vi "1022test.vi"() -> ()   [LabVIEW 2019]
panel:
  out "Read Buffer":string
  in  "Timeout":u32=1000
  in  "Remote Mode":u16(ring) items=["USB", "RS232", "GPIB"]
  out "Serial Versions":string
  in  "Baud rate (921600)":u32=921600
  in  "VISA resource name":refnum<visa-resource-name>
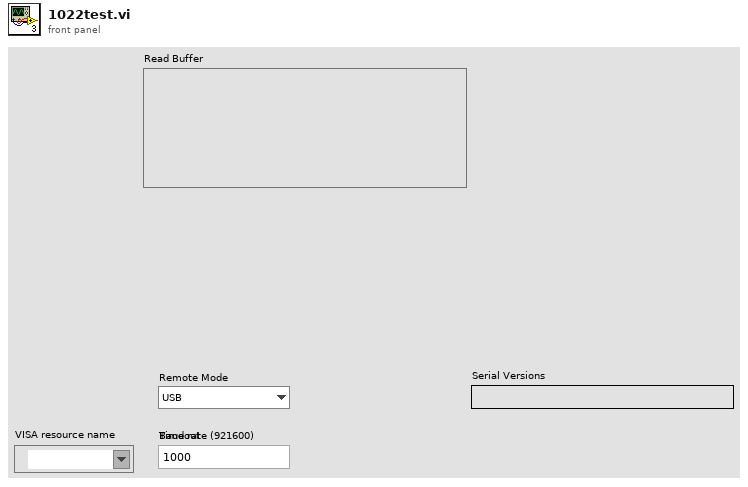
[diagram p1: front panel]
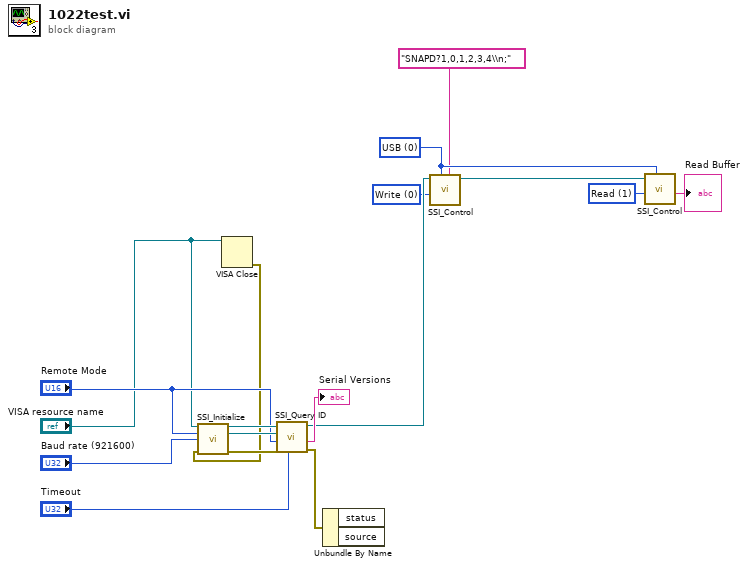
[diagram p0: block diagram]
diagram:
  w3 = u16 1 items=["Write", "Read"] ("Control")
  w4 = u16 0 items=["Write", "Read"] ("Control")
  w5 = u16 0 items=["USB", "RS232", "GPIB", "Ethernet"] ("Remote Mode")
  n1 = VISA Close(VISA resource name="VISA resource name") -> (error out=w8:errorcluster)  [unwired: 1 in]
  n2 = call "SSI_Initialize.vi"("VISA resource name"="VISA resource name", "Remote Mode"="Remote Mode", "baud rate (921600)"="Baud rate (921600)", "error in (no error)"=w8) -> ("VISA resource name out"=w16:refnum<visa-resource-name>, "connection ID(Ethernet)"=w15:refnum<k5>, "error out"=w14:errorcluster)  [unwired: 9 in]
  n3 = call "SSI_Query ID.vi"("Timeout"="Timeout", "Error in (no error)"=w14, "Remote Mode"="Remote Mode", "Connection ID in"=w15, "VISA resource name"=w16) -> ("Error out"=w11:errorcluster, "Read Buffer"=→"Serial Versions":string, "VISA resource  out"=w7:refnum<visa-resource-name>)  [unwired: 3 in, 1 out]
  n4 = Unbundle By Name(w11) -> ()  [unwired: 2 out]
  n5 = call "SSI_Control.vi"("Write Buffer"="SNAPD?1,0,1,2,3,4\\n;", "Remote Mode"=w5, "Control"=w4, "VISA resource name"=w7) -> ("VISA resource  out"=w6:refnum<visa-resource-name>)  [unwired: 4 in, 3 out]
  n6 = call "SSI_Control.vi"("Remote Mode"=w5, "Control"=w3, "VISA resource name"=w6) -> ("Read Buffer"=→"Read Buffer":string)  [unwired: 5 in, 3 out]
